vi "ROI_sum.vi"(9 "unsigned 64bit integer":u64[][](array[numeric]), 10 "Background Regions (Left, Top, Right, Bottom)":i32[][](array[numeric]), 11 "Regions of Interest (Left, Top, Right, Bottom)":i32[][](array[numeric])) -> (3 "Array of ROI sums":dbl[](array[numeric]))   [LabVIEW 2013]
panel:
  out "Array":dbl[](array[numeric])
  out "Numeric":dbl
  out "subarray":u64[][](array[numeric])
  out "x-y 3":i32
  out "x-y 2":i32
  out "sum 2":dbl
  out "x-y":dbl[][](array[numeric])
  out "unsigned 64bit integer 2":u64[][](array[numeric])
  out "sum":i32
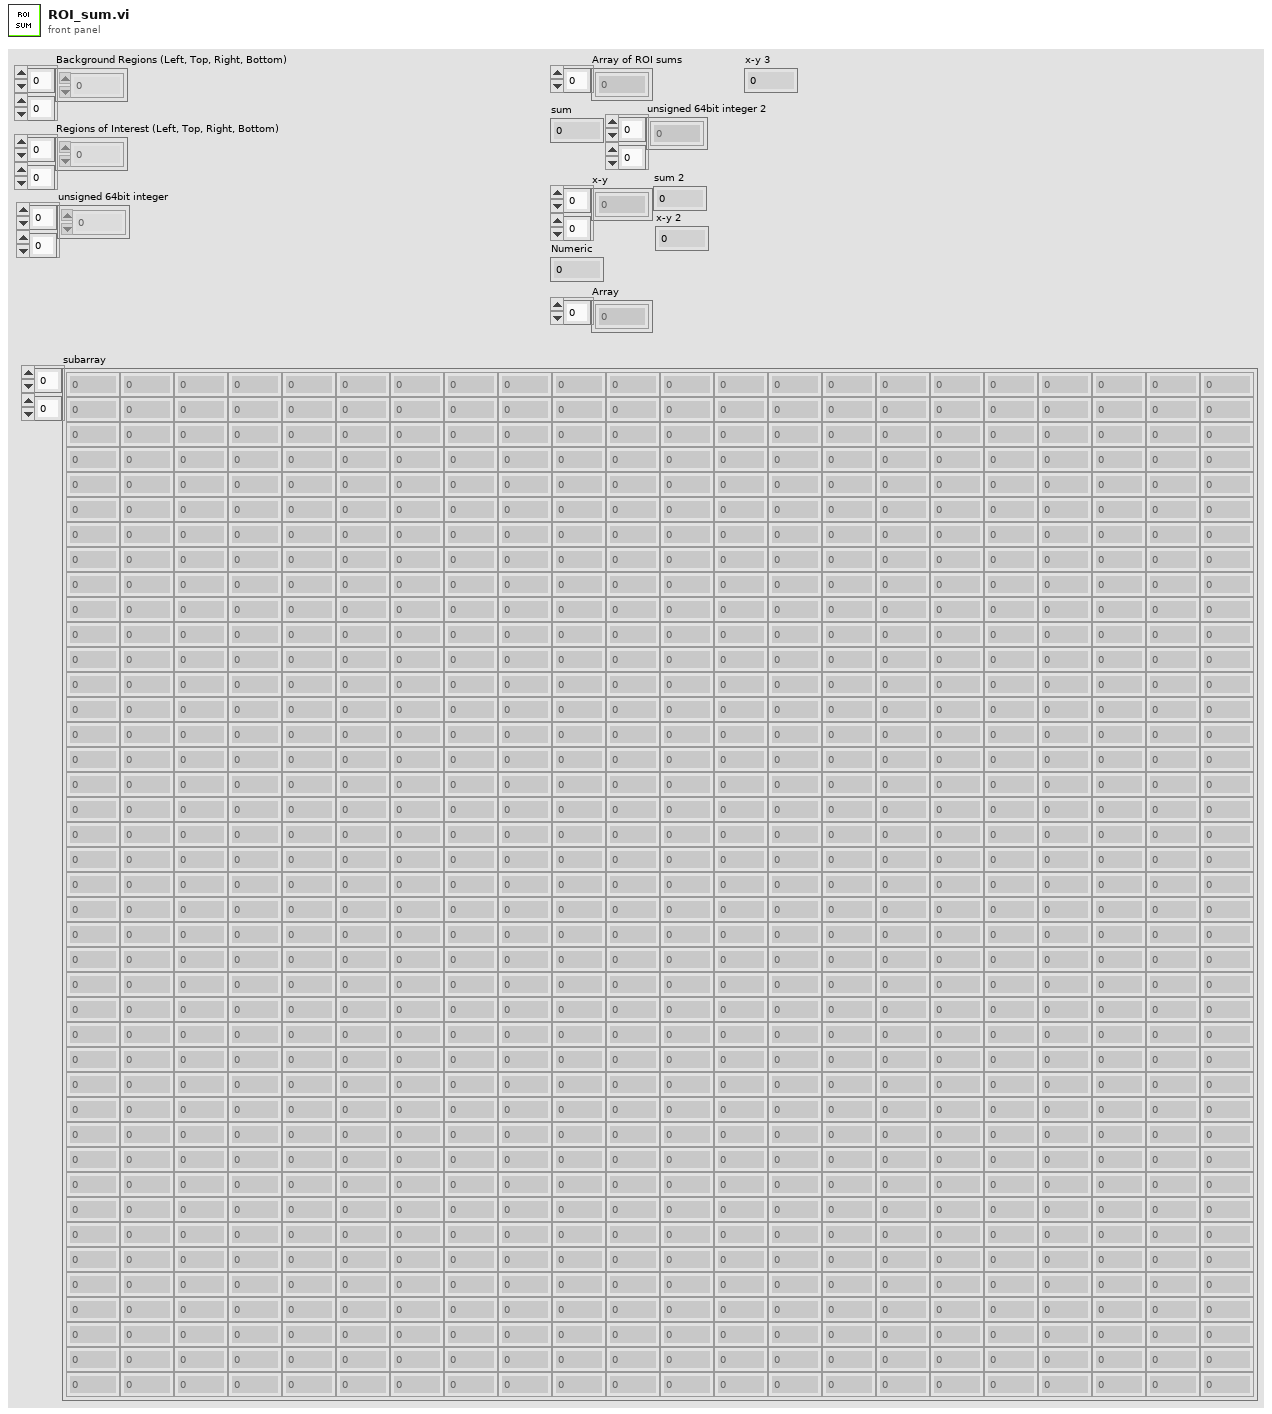
[diagram p1: front panel]
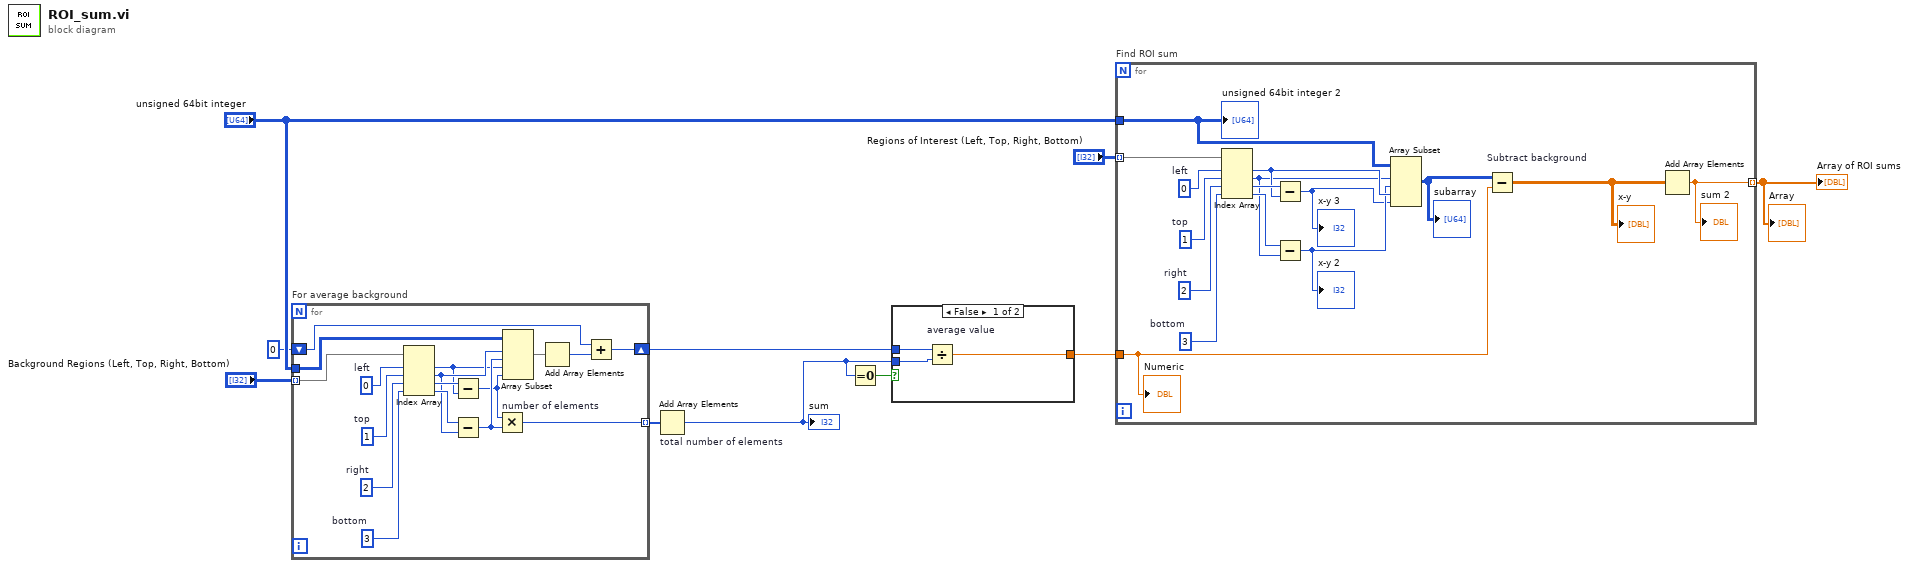
[diagram p0: block diagram]
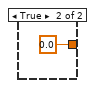
[diagram p2: hidden frame]
diagram:
  n1 = for "For average background" {
    tunnel: "unsigned 64bit integer" -> [w20]
    tunnel: "Background Regions (Left, Top, Right, Bottom)" -> [w27] mode=indexing
    tunnel: [w15] -> w7 mode=indexing
    shift-right: [w16] -> w2
    shift-left: u64 0 -> [w18]
    w23 = 3  # bottom
    w24 = 2  # right
    w25 = 1  # top
    w26 = 0  # left
    n2 = Index Array(array=w27, index #1=w26, index #2=w25, index #3=w24, index #4=w23) -> (element #1=w11:i32, element #2=w13:i32, element #3=w21:i32, element #4=w22:i32)
    n3 = Subtract(x=w21, y=w11) -> (x-y=w12:i32)
    n4 = Subtract(x=w22, y=w13) -> (x-y=w14:i32)
    n5 = Multiply "number of elements"(x=w12, y=w14) -> (x*y=w15:i32)
    n6 = Array Subset(array=w20, index (row)=w13, length (row)=w14, index (col)=w11, length (col)=w12) -> (w19:u64[][])
    n7 = Add Array Elements(numeric array=w19) -> (sum=w17:u64)
    n8 = Add(x=w18, y=w17) -> (x+y=w16:u64)
  }
  n9 = Add Array Elements "total number of elements"(numeric array=w7) -> (sum=w3:i32)
  "sum" <- w3
  n10 = Equal To 0?(x=w3) -> (x = 0?=w4:bool)
  n11 = case shown="False" w4 {
    tunnel: w3 -> [w30 _]
    tunnel: w2 -> [w29 _]
    tunnel: [w28 0.0] -> w1
    frame False {
      n12 = Divide "average value"(x=w29, y=w30) -> (x/y=w28:dbl)
    }
    frame True {
    }
  }
  n13 = for "Find ROI sum" {
    tunnel: "unsigned 64bit integer" -> [w40]
    tunnel: "Regions of Interest (Left, Top, Right, Bottom)" -> [w47] mode=indexing
    tunnel: w1 -> [w38]
    tunnel: [w36] -> w6 mode=indexing
    w43 = 3  # bottom
    w44 = 2  # right
    w45 = 1  # top
    w46 = 0  # left
    n14 = Index Array(array=w47, index #1=w46, index #2=w45, index #3=w44, index #4=w43) -> (element #1=w35:i32, element #2=w34:i32, element #3=w41:i32, element #4=w42:i32)
    n15 = Subtract(x=w41, y=w35) -> (x-y=w32:i32)
    "x-y 3" <- w32
    n16 = Subtract(x=w42, y=w34) -> (x-y=w33:i32)
    "x-y 2" <- w33
    n17 = Array Subset(array=w40, index (row)=w34, length (row)=w33, index (col)=w35, length (col)=w32) -> (w39:u64[][])
    "subarray" <- w39
    n18 = Subtract "Subtract background"(x=w39, y=w38) -> (x-y=w37:dbl[][])
    "x-y" <- w37
    n19 = Add Array Elements(numeric array=w37) -> (sum=w36:dbl)
    "sum 2" <- w36
    "unsigned 64bit integer 2" <- w40
    "Numeric" <- w38
  }
  "Array of ROI sums" <- w6
  "Array" <- w6
